vi "SIMUSIN.vi"() -> ()   [LabVIEW 2017]
uses:
  Typedefs/Tipo_TipoSinalSimulado.ctl
  Typedefs/Tipo_DadosCanal.ctl
  Typedefs/Tipo_BlocoSinais.ctl
  Typedefs/Tipo_ConfigSistema.ctl
  Typedefs/Tipo_ParamsRuido.ctl
  <vilib>/NI/STM/SubVIs/MetaDataElement.ctl
  <vilib>/NI/STM/Connection Manager/TCP/TCP Connection Method.ctl
  <vilib>/NI/STM/TCP/TCP Read Options.ctl
  Typedefs/Tipo_PoolComando.ctl
  <vilib>/NI/STM/TCP/Write Meta Data (TCP Ref).vi
  <vilib>/NI/STM/TCP/Write Meta Data (TCP Clst).vi
  <vilib>/NI/STM/TCP/Read Message (TCP).vi
  <vilib>/NI/STM/TCP/Write Message (TCP).vi
  <vilib>/NI/STM/TCP/TCP Connection Info.ctl
  <vilib>/NI/STM/NI STM.lvlib
panel:
  out "BlocoBaixaEnviado":i32
  out "SinaisBaixa":waveform(dbl)[](array[waveform])
  in  "ParamsCanalCopiado":variant
  out "DadosEstaticos":dbl[](array[numeric])
  in  "Tab Control":enum32{"Dinâmicos", "Estáticos"}(tab)
  in  "TxAmostragemBaixa":dbl=300.0 caption="Tx. Baixa (Hz):" min=50.0 max=50000.0
  out "NumConexoes":i32 caption="Num. Conexões"
  in  "CopiarCanal":bool
  in  "ColarCanal":bool
  in  "Canais":i32[](listbox)
  out "Índice":i32
  in  "Nome":string
  in  "Tipo":T1
  in  "NovoCanal":bool
  in  "AtualizarCanal":bool
  in  "ExcluirCanal":bool
  out "Frequência":cluster{"f0":dbl, "df":dbl, "magnitude":dbl[]}[](graph)
  out "Tempo":waveform(dbl)[](graph)
  in  "TxAmostragem":dbl=300.0 caption="Tx. Amostragem (Hz):" min=50.0 max=100000.0
  in  "Porta":u16=2099
  out "NumBloco":i32 caption="Bloco:"
  in  "SobeCanal":bool
  in  "DesceCanal":bool
  in  "Habilitar":bool caption="Habilitado"
  in  "Vizualizar Baixa":bool
  in  "Ver Fase":bool
  in  "RemoverPonto":bool
  in  "InserirPonto":bool
  in  "Sinais Estáticos":i32(listbox)
  in  "DesceCanalEstatico":bool
  in  "SobeCanalEstatico":bool
  out "Sinais":waveform(dbl)[](array[waveform])
  in  "ResetCanais":bool
  in  "Saiu?":bool
  in  "DadosCanais":T2[](array[typedef])
  # "SimuSinC - Simulador de Sinais"
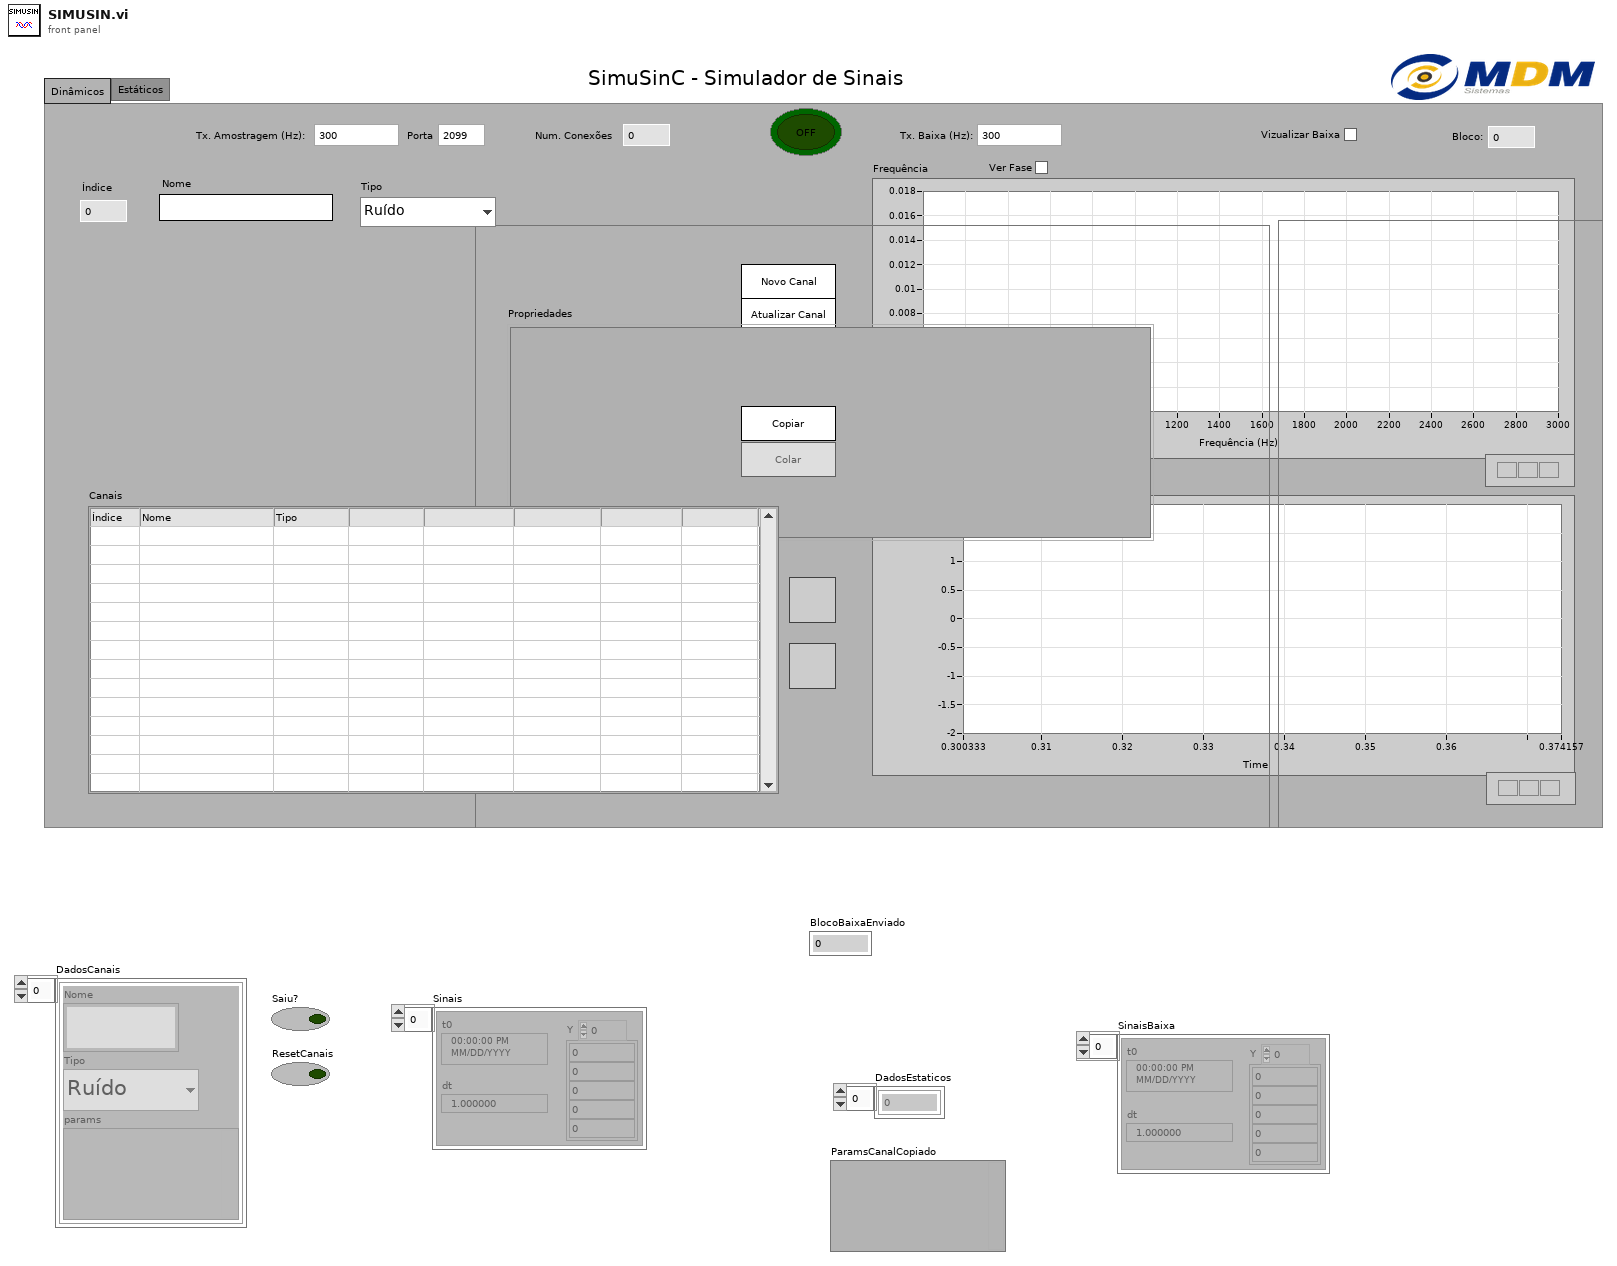
[diagram p1: front panel]
types:
  T1 = typedef "Tipo_TipoSinalSimulado.ctl" = enum16{"Ruído", "Fasor", "Senóide", "Composto", "AM", "Proximidade", "Entreferro"}
  T2 = typedef "Tipo_DadosCanal.ctl" = cluster{"Nome":string, "Tipo":T1, "params":variant}
  T3 = typedef "Tipo_BlocoSinais.ctl" = cluster{"SinaisAlta":waveform(dbl)[], "SinaisBaixa":waveform(dbl)[], "NumBloco":i32}
  T4 = enum8{"Enabled", "Disabled", "Disabled and Grayed Out"}
  T5 = typedef "Tipo_ConfigSistema.ctl" = cluster{"TxAmostragem":dbl, "Porta":u16, "TxAmostragemBaixa":dbl}
  T6 = typedef "Tipo_ParamsRuido.ctl" = cluster{"Amplitude":dbl, "Banda: ":bool, "Freq. Inferior":dbl, "Freq. Superior":dbl}
  T7 = typedef "FileVersionInformation.ctl" = cluster{"FileVersion":string, "ProductName":string, "InternalName":string, "CompanyName":string, "LegalCopyright":string, "FileDescription":string}
  T8 = typedef "LVPoint32TypeDef.ctl" = cluster{"Horizontal":i32, "Vertical":i32}
  T9 = typedef "LVRowAndColumnTypeDef.ctl" = cluster{"Row":i32, "Column":i32}
  T10 = typedef "NI STM.lvlib/TCP Connection Info.ctl" = cluster{"connection ID":refnum<k5>, "meta data":T11[]}
  T11 = typedef "NI STM.lvlib/MetaDataElement.ctl" = string
  T12 = typedef "Tipo_PoolComando.ctl" = enum16{"Indefinido", "ProximoBlocoAlta", "ProximoBlocoBaixa"}
  T13 = typedef "NI STM.lvlib/TCP Connection Method.ctl" = enum16{"Initialize", "Add Connection", "Set Properties", "Get Connection(s)", "Remove Connection", "Remove All Connections", "Get Connection Count"}
  T14 = typedef "NI STM.lvlib/TCP Read Options.ctl" = cluster{"ignore timeout error":bool, "timeout ms (1000)":i32}
  T15 = typedef "Tipo_PacoteModuloCRIO.ctl" = cluster{"modulo":T16, "sinais":cluster{"dados":sgl[]}[], "numBloco":i32}
  T16 = typedef "Tipo_moduloCRIO.ctl" = cluster{"nome":string, "modelo":string, "slot":i32, "numCanais":i32, "canaisInativos":i32[], "sensores":string[], "TaxaAquisicao":dbl}
  T17 = cluster{waveform(dbl)[], "SinaisBaixa":waveform(dbl)[], i32}
  T18 = enum32{"invalid app kind", "Development System", "Run Time System", "Student Edition", "Embedded LabVIEW", "Evaluation", "Custom"}
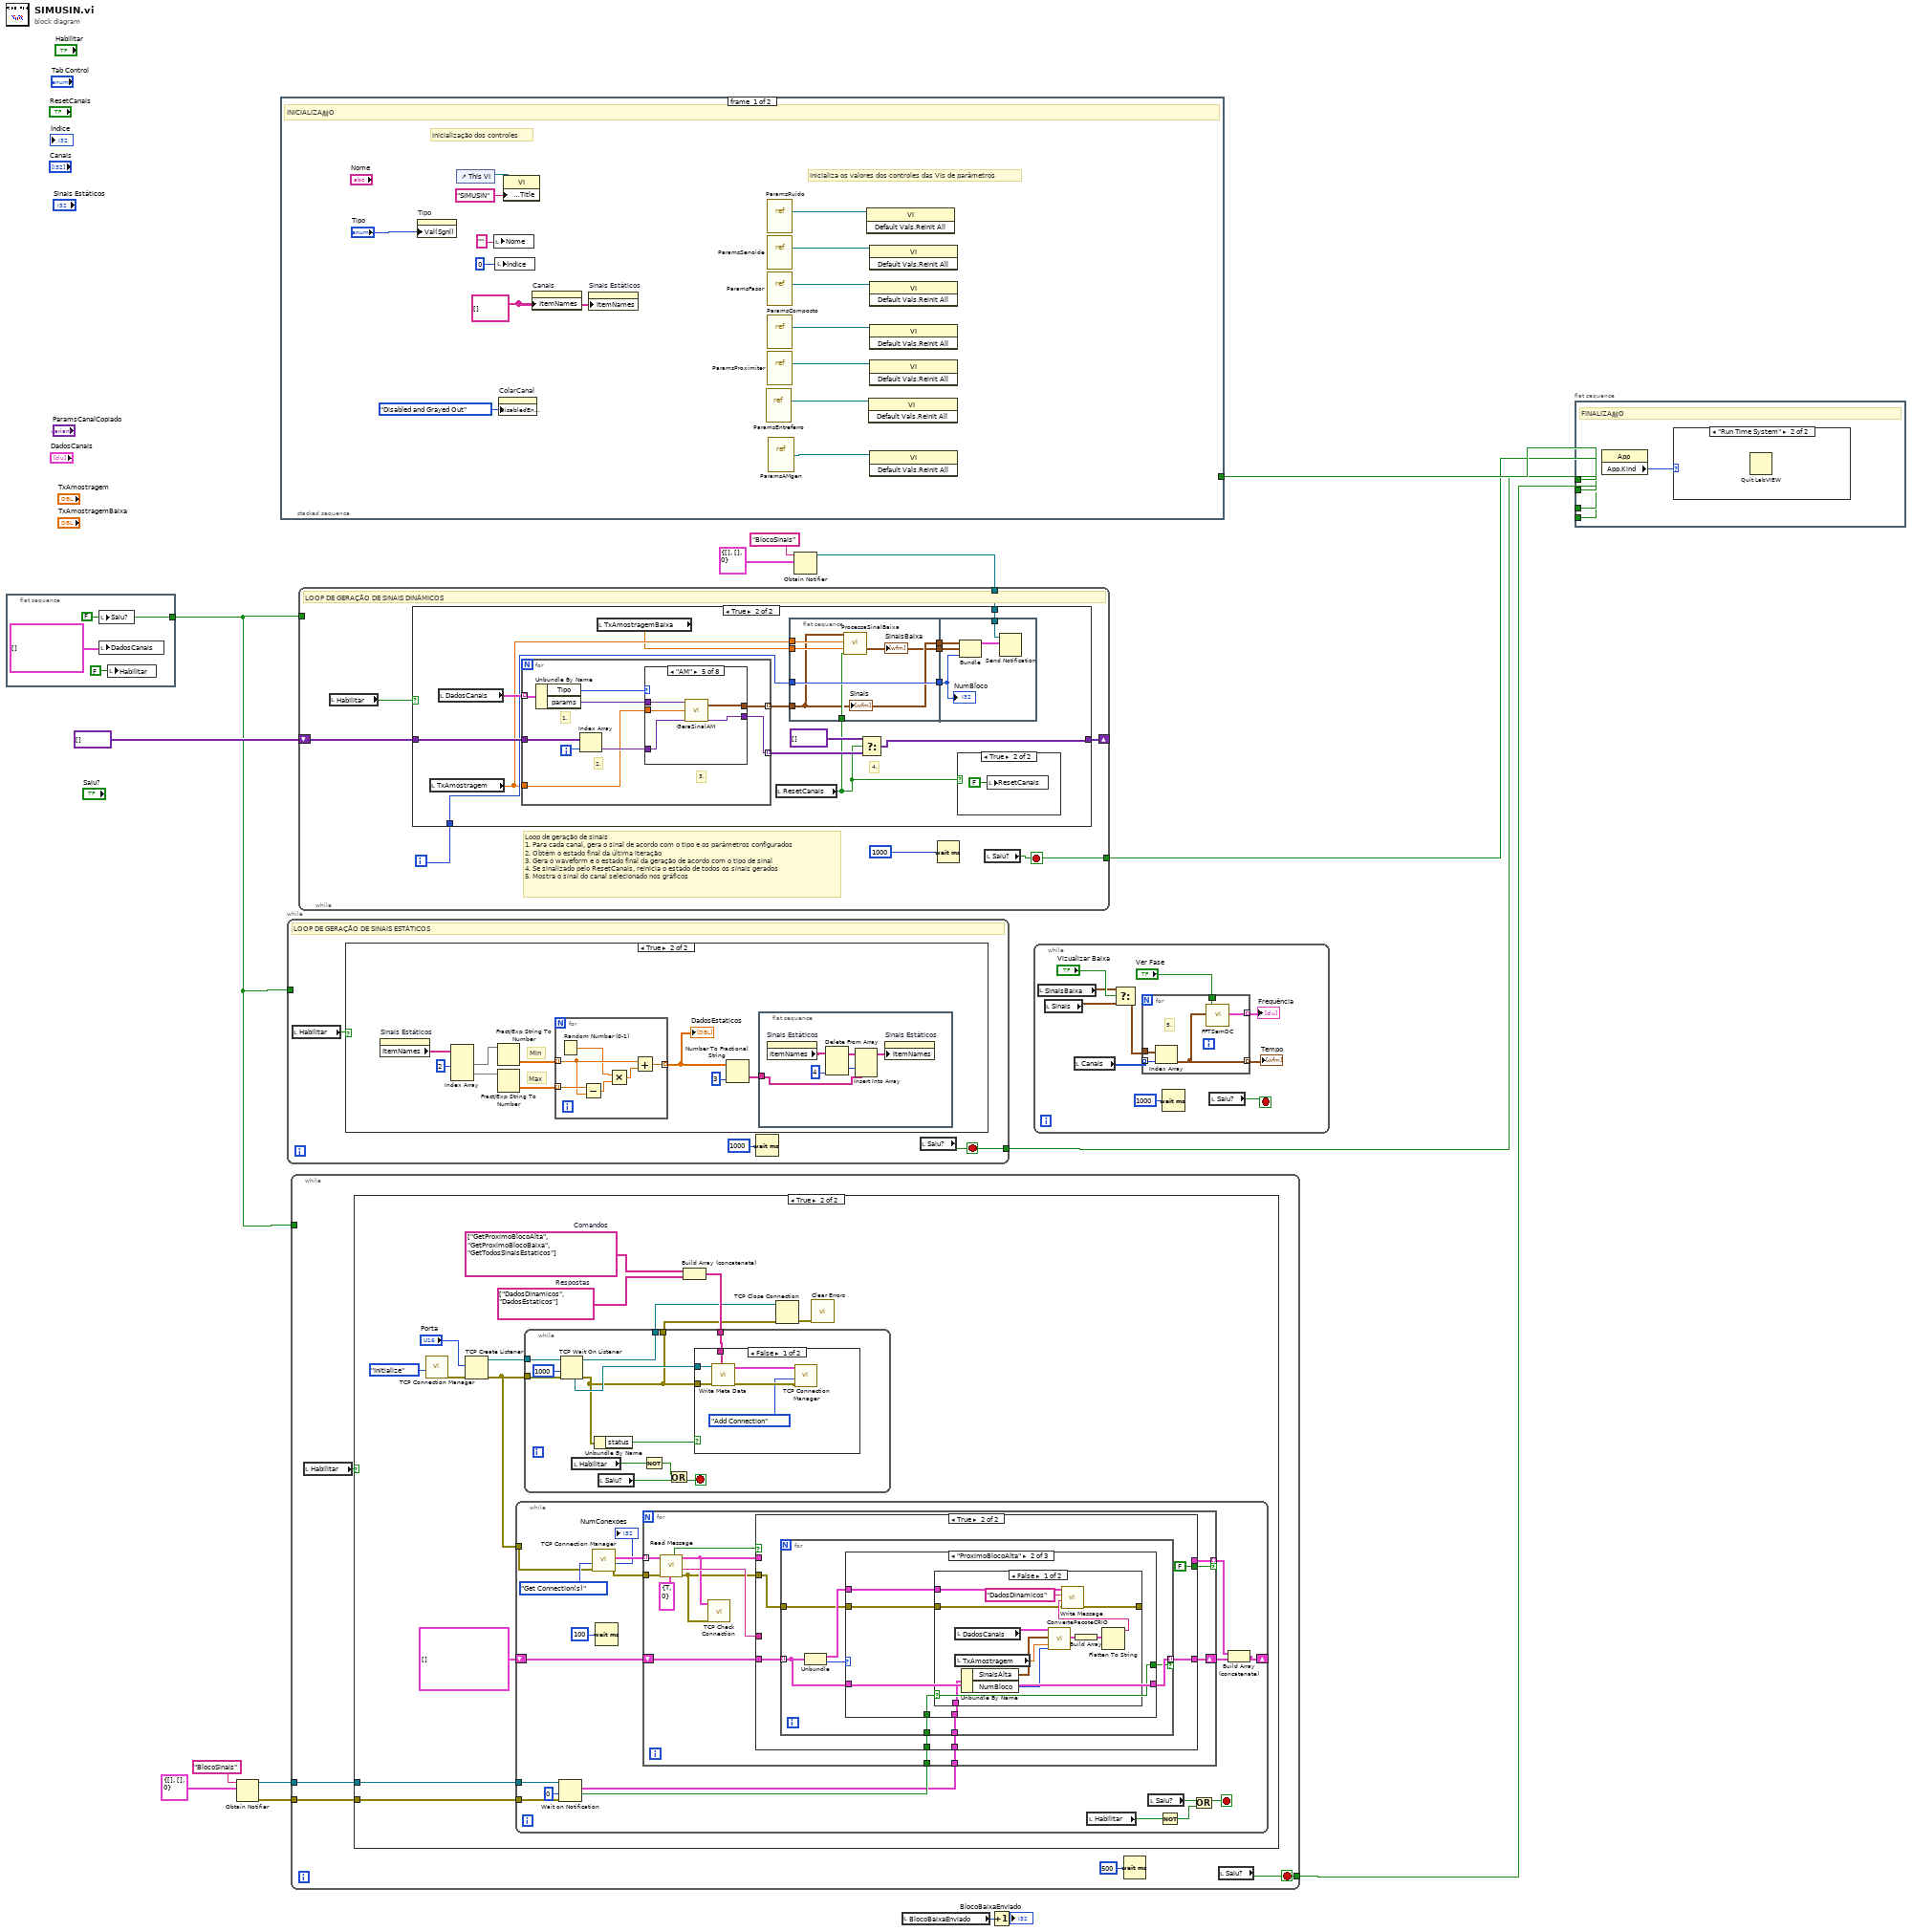
[diagram p0: block diagram]
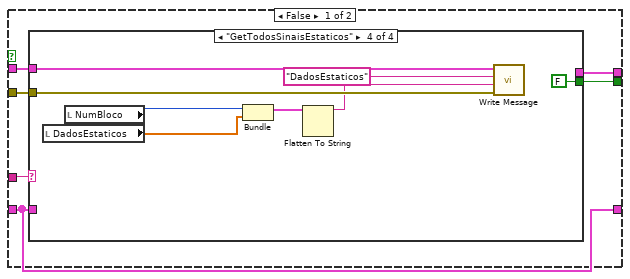
[diagram p3: hidden frame]
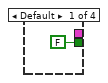
[diagram p4: hidden frame]
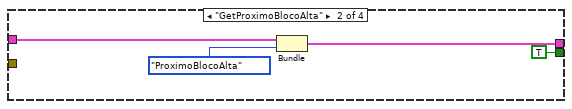
[diagram p5: hidden frame]
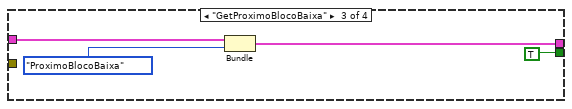
[diagram p6: hidden frame]
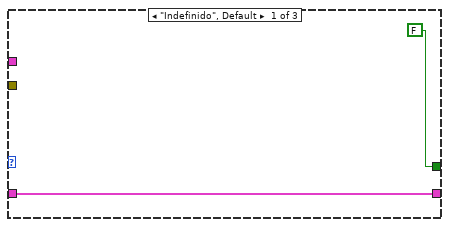
[diagram p7: hidden frame]
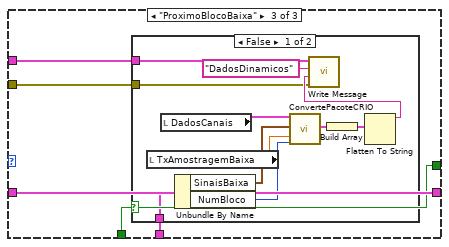
[diagram p9: hidden frame]
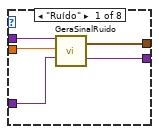
[diagram p16: hidden frame]
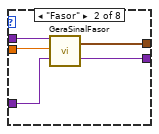
[diagram p17: hidden frame]
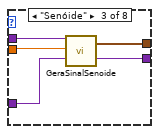
[diagram p18: hidden frame]
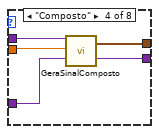
[diagram p19: hidden frame]
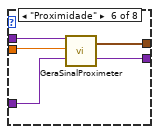
[diagram p20: hidden frame]
diagram:
  n1 = flat-sequence {
    tunnel: [w18] -> w10
    frame #0 {
      w18 = FALSE ("Saiu?")
      n2 = local write "Saiu?"(w18) -> ()
      n3 = local write "DadosCanais"(T2[] [] ("DadosCanais")) -> ()
      n4 = local write "Habilitar"(FALSE ("Habilitar")) -> ()
    }
  }
  n5 = Obtain Notifier(name (unnamed)="BlocoSinais", notification data type=T3 {"SinaisAlta"=[], "SinaisBaixa"=[], "NumBloco"=0} ("output cluster")) -> (notifier out=w4:refnum<notifier>, error out=w3:errorcluster)  [unwired: 2 in, 1 out]
  n6 = stacked-sequence {
    tunnel: [_ w33] -> w14
    frame #0 {
      w26 = string[][] [] ("Item Names")
      # "Inicializa os valores dos controles das VIs de parâmetros"
      # "Inicialização dos controles"
      # "INICIALIZA敲O"
      n7 = property on="Tipo" class="Enum (strict)"("Val(Sgnl)"="Tipo") -> ()  [unwired: 2 in, 2 out]
      n8 = control-ref of="This VI"() -> (w25:refnum<vi>)
      n9 = local write "Nome"("" ("Nome")) -> ()
      n10 = local write "Índice"(0 ("Índice")) -> ()
      n11 = property on="ColarCanal" class="Bool"("DisabledEnum"=T4."Disabled and Grayed Out" ("Disabled")) -> ()  [unwired: 2 in, 2 out]
      n12 = property class="VI"(reference=w25, "Front Panel.Title"="SIMUSIN" ("Front Panel Window:Title")) -> ()  [unwired: 1 in, 2 out]
      n13 = property on="Canais" class="MCListbox (strict)"("ItemNames"=w26) -> ()  [unwired: 2 in, 2 out]
      n14 = property on="Sinais Estáticos" class="MCListbox (strict)"("ItemNames"=w26) -> ()  [unwired: 2 in, 2 out]
      n15 = vi-ref "ParamsEntreferro.vi"() -> (w20:refnum<vi>)
      n16 = vi-ref "ParamsRuido.vi"() -> (w30:refnum<vi>)
      n17 = vi-ref "ParamsSenoide.vi"() -> (w29:refnum<vi>)
      n18 = vi-ref "ParamsFasor.vi"() -> (w28:refnum<vi>)
      n19 = vi-ref "ParamsComposto.vi"() -> (w21:refnum<vi>)
      n20 = vi-ref "ParamsProximiter.vi"() -> (w22:refnum<vi>)
      n21 = vi-ref "ParamsAMgen.vi"() -> (w19:refnum<vi>)
      n22 = invoke class="VI" method="Default Vals.Reinit All"(reference=w30) -> ()  [unwired: 2 in, 3 out]
      n23 = invoke class="VI" method="Default Vals.Reinit All"(reference=w20) -> ()  [unwired: 2 in, 3 out]
      n24 = invoke class="VI" method="Default Vals.Reinit All"(reference=w29) -> ()  [unwired: 2 in, 3 out]
      n25 = invoke class="VI" method="Default Vals.Reinit All"(reference=w28) -> ()  [unwired: 2 in, 3 out]
      n26 = invoke class="VI" method="Default Vals.Reinit All"(reference=w21) -> ()  [unwired: 2 in, 3 out]
      n27 = invoke class="VI" method="Default Vals.Reinit All"(reference=w22) -> ()  [unwired: 2 in, 3 out]
      n28 = invoke class="VI" method="Default Vals.Reinit All"(reference=w19) -> ()  [unwired: 2 in, 3 out]
    }
    frame #1 {
      # "LOOP DE INTERFACE"
      n29 = while {
        tunnel: [w34] -> w33
        stop <- w34 stop-if-true
        # "LOOP DE INTERFACE"
        n30 = event shown="[3] \"Tipo\": Value Change" {
          selector: _ -> [_ _ _ _ _ _ _ _ _ _ _ _ _ _ _ _ _ _ _]
          dyn-events: _ -> [_ _ _ _ _ _ _ _ _ _ _ _ _ _ _ _ _ _ _]
          timeout: 500 -> [_ _ _ _ _ _ _ _ _ _ _ _ _ _ _ _ _ _ _]
          tunnel: [_ _ w49 _ _ _ _ _ _ _ _ _ _ _ _ _ _ _ _] -> w34
          event Timeout {
            n31 = event-data() -> ()  [unwired: 1 in, 2 out]
          }
          event "Canais": Value Change {
            # "2."
            # "1."
            # "Evento: Troca de canal selecionado\n1. Obtém os dados do novo canal selecionado\n2. Muda o valor do tipo de sinal sinalizando o evento para atualizar o VI de parâmetros sendo mostrado\n3. Se for uma seleção válida, atualiza os parâmetros da VI apropriada\n4. Reinicia o chart do sinal no tempo"
            n32 = event-data() -> ("NewVal"=w41:i32[])  [unwired: 1 in, 4 out]
            n33 = Index Array(array=w41) -> (element=w36:i32)  [unwired: 1 in]
            n34 = local read "DadosCanais"() -> (w39:T2[])
            n35 = local write "Índice"(w36) -> ()
            n36 = Index Array(array=w39, index=w36) -> (element=w43:T2)
            n37 = Unbundle By Name(w43) -> ("Nome"=w42:string, "Tipo"=w37:T1, "params"=w40:variant)
            n38 = Array Size(array=w39) -> (size(s)=w38:i32)
            n39 = property on="Tipo" class="Enum (strict)"("Val(Sgnl)"=w37) -> ()  [unwired: 2 in, 2 out]
            n40 = local write "Nome"(w42) -> ()
            n41 = case shown="Default" w38 {
              tunnel: w40 -> [_ w46]
              tunnel: w37 -> [_ w45]
              frame 0 {
              }
              frame Default {
                # "3."
                n42 = call "GetVIParam.vi"("Tipo"=w45) -> ("vi reference"=w44:refnum<vi>)  [unwired: 18 in]
                n43 = call "AtualizaPainel.vi"("VI in"=w44, "Init"=TRUE, "ParamsIn"=w46) -> ()  [unwired: 16 in, 1 out]
              }
            }
          }
          event Menu Selection (User) {
            # "Processa eventos do menu superior"
            n44 = event-data() -> ("MenuRef"=w48:refnum<k9>, "ItemTag"=w50:string)  [unwired: 1 in, 4 out]
            n45 = case shown="\"ImportarDinamicos\"" w50 {
              selector: w50 -> [_ _ _ _ _ _ _ _ w170]
              tunnel: [FALSE TRUE _ FALSE FALSE FALSE FALSE FALSE _] -> w49
              tunnel: w48 -> [_ _ _ _ _ _ _ _ w171]
              frame Default {
              }
              frame "Sair" {
                # "Evento Sair"
              }
              frame "Sobre" {
                n46 = property class="App"() -> ("App.Dir"=w63:path, "App.Name"=w62:string)  [unwired: 2 in, 2 out]
                n47 = Build Path(base path=w63, name or relative path=w62) -> (appended path=w61:path)
                n48 = call <vilib>:"FileVersionInfo.vi"("Application Path in"=w61) -> ("FileVersionInfo Out"=w60:T7)  [unwired: 7 in, 3 out]
                n49 = Unbundle By Name(w60) -> ("ProductName"=w58:string, "FileVersion"=w57:string, "CompanyName"=w56:string, "LegalCopyright"=w55:string, "FileDescription"=w54:string)
                n50 = Format Into String(format string="%s versão %s\n%s\n%s\n%s", w58, w57, w56, w55, w54) -> (resulting string=w53:string)  [unwired: 2 in, 1 out]
                n51 = One Button Dialog(message=w53) -> ()  [unwired: 1 in, 1 out]
              }
              frame "SalvarConfig" {
                n52 = local read "TxAmostragemBaixa"() -> (w64:dbl)
                n53 = local read "TxAmostragem"() -> (w66:dbl)
                n54 = local read "Porta"() -> (w65:u16)
                n55 = call "File Dialog"("prompt"="Salvar arquivo de configuração", "pattern (all files)"="*.cfg", "pattern label"="Configuração de canais") -> ("selected path"=w73:path, "cancelled"=w71:bool, "error out"=w70:errorcluster)  [unwired: 9 in, 1 out]
                n56 = Bundle(cluster=T5 {"TxAmostragem"=0.0, "Porta"=0, "TxAmostragemBaixa"=0.0} ("output cluster"), "TxAmostragem"=w66, "Porta"=w65, "TxAmostragemBaixa"=w64) -> (w68:T5)
                n57 = case shown="False" w71 {
                  tunnel: w73 -> [w79 _]
                  tunnel: w70 -> [w77 _]
                  tunnel: w68 -> [w76 _]
                  frame False {
                    # "Salva os dados dos canais em arquivo"
                    n58 = local read "DadosCanais"() -> (w81:T2[])
                    n59 = property on="Sinais Estáticos" class="MCListbox (strict)"() -> ("ItemNames"=w80:string[][])  [unwired: 2 in, 2 out]
                    n60 = call "SalvarConfig.vi"("caminho in"=w79, "CanaisDinamicos"=w81, "CanaisEstaticos"=w80, "ConfigSistema"=w76, "error in"=w77) -> ("caminho out"=w78:path, "error out"=w82:errorcluster)  [unwired: 13 in]
                    n61 = case shown="No Error" w82 {
                      selector: w82 -> [_ w88]
                      tunnel: w78 -> [w83 _]
                      frame No Error {
                        n62 = Format Into String(format string="SIMUSIN (%s)", w83) -> (resulting string=w84:string)  [unwired: 2 in, 1 out]
                        n63 = control-ref of="This VI"() -> (w85:refnum<vi>)
                        n64 = property class="VI"(reference=w85, "Front Panel.Title"=w84) -> ()  [unwired: 1 in, 2 out]
                        n65 = One Button Dialog(message="Configuração salva com sucesso!") -> ()  [unwired: 1 in, 1 out]
                      }
                      frame Error {
                        n66 = call <vilib>:"Simple Error Handler.vi"("error in (no error)"=w88) -> ()  [unwired: 4 in, 5 out]
                      }
                    }
                  }
                  frame True {
                  }
                }
              }
              frame "CarregarConfig" {
                n67 = call "File Dialog2"("prompt"="Carregar arquivo de configuração", "pattern (all files)"="*.cfg", "pattern label"="Configuração de canais") -> ("selected path"=w92:path, "cancelled"=w91:bool, "error out"=w90:errorcluster)  [unwired: 9 in, 1 out]
                n68 = case shown="False" w91 {
                  tunnel: w92 -> [w109 _]
                  tunnel: w90 -> [w108 _]
                  frame False {
                    # "Carrega os dados dos canais\ndo arquivo"
                    n69 = call "CarregarConfig.vi"("caminho in"=w109, "error in (no error)"=w108) -> ("caminho out"=w106:path, "DadosCanais"=w110:T2[], "Estaticos"=w107:string[][], "ConfigSistema"=w105:T5, "error out"=w96:errorcluster)  [unwired: 13 in]
                    n70 = call <vilib>:"Simple Error Handler.vi"("error in (no error)"=w96) -> ()  [unwired: 4 in, 5 out]
                    n71 = Unbundle(w105) -> ("TxAmostragem"=w99:dbl, "Porta"=w98:u16, "TxAmostragemBaixa"=w97:dbl)
                    n72 = property on="Sinais Estáticos" class="MCListbox (strict)"("ItemNames"=w107) -> ()  [unwired: 2 in, 2 out]
                    n73 = Format Into String(format string="SIMUSIN (%s)", w106) -> (resulting string=w100:string)  [unwired: 2 in, 1 out]
                    n74 = local write "Porta"(w98) -> ()
                    n75 = local write "TxAmostragemBaixa"(w97) -> ()
                    n76 = local write "TxAmostragem"(w99) -> ()
                    n77 = call "PopulaListaCanais.vi"("DadosCanais"=w110) -> ("Strings"=w103:string[][])  [unwired: 18 in]
                    n78 = control-ref of="This VI"() -> (w102:refnum<vi>)
                    n79 = property on="Canais" class="MCListbox (strict)"("ItemNames"=w103) -> ()  [unwired: 2 in, 2 out]
                    n80 = local write "DadosCanais"(w110) -> ()
                    n81 = property class="VI"(reference=w102, "Front Panel.Title"=w100) -> ()  [unwired: 1 in, 2 out]
                    n82 = One Button Dialog(message="Configuração carregada com sucesso!") -> ()  [unwired: 1 in, 1 out]
                  }
                  frame True {
                  }
                }
              }
              frame "NovaConfig" {
                n83 = Two Button Dialog(message="Alterações não salvas na configuração atual\nserão perdidas. Deseja continuar? ", 1:"Não" ("T button name (\"OK\")"), 2:"Sim" ("T button name (\"OK\")")) -> (T button?=w112:bool)
                n84 = case shown="True" w112 {
                  frame False {
                  }
                  frame True {
                    n85 = local write "Nome"("" ("Nome")) -> ()
                    n86 = local write "Índice"(0 ("Índice")) -> ()
                    n87 = property on="Canais" class="MCListbox (strict)"("ItemNames"=string[][] [] ("Item Names")) -> ()  [unwired: 2 in, 2 out]
                    n88 = local write "DadosCanais"(T2[] [] ("DadosCanais")) -> ()
                  }
                }
              }
              frame "ImportarEstaticos" {
                n89 = call "File Dialog3"("pattern (all files)"="*.csv", "pattern label"="Arquivo CSV") -> ("selected path"=w121:path, "cancelled"=w122:bool, "error out"=w120:errorcluster)  [unwired: 10 in, 1 out]
                n90 = case shown="False" w122 {
                  tunnel: w121 -> [w141 _]
                  tunnel: w120 -> [w128 _]
                  frame False {
                    n91 = Read from Text File(file (use dialog)=w141, error in=w128) -> (text=w140:string, error out=w127:errorcluster)  [unwired: 2 in, 2 out]
                    n92 = Spreadsheet String To Array(delimiter (Tab)=";", format string="%s", spreadsheet string=w140, array type (2D Dbl)=string[][] []) -> (array=w133:string[][])
                    n93 = Array Size(array=w133) -> (size(s)=w136:i32[])
                    n94 = Index Array(array=w136) -> (element=w134:i32)  [unwired: 1 in]
                    n95 = Initialize Array("", w134) -> (w131:string[])
                    n96 = Insert Into Array(array=w133, index (col)=0 ("disabled index (col)"), new element=w131) -> (w130:string[][])  [unwired: 1 in]
                    n97 = call "IndexaEstaticos.vi"("Strings"=w130) -> ("StringsIndexadas"=w129:string[][])  [unwired: 18 in]
                    n98 = property on="Sinais Estáticos" class="MCListbox (strict)"(error in=w127, "ItemNames"=w129) -> (error out=w126:errorcluster)  [unwired: 1 in, 1 out]
                    n99 = case shown="No Error" w126 {
                      selector: w126 -> [_ w143]
                      frame No Error {
                        n100 = One Button Dialog(message="Arquivo importado com sucesso!") -> ()  [unwired: 1 in, 1 out]
                      }
                      frame Error {
                        n101 = call <vilib>:"Simple Error Handler.vi"("error in (no error)"=w143) -> ()  [unwired: 4 in, 5 out]
                      }
                    }
                  }
                  frame True {
                  }
                }
              }
              frame "ImportarDinamicos" {
                n102 = call "File Dialog4"("pattern (all files)"="*.csv", "pattern label"="Arquivo CSV") -> ("selected path"=w145:path, "cancelled"=w146:bool, "error out"=w144:errorcluster)  [unwired: 10 in, 1 out]
                n103 = case shown="False" w146 {
                  tunnel: w145 -> [w160 _]
                  tunnel: w144 -> [w155 _]
                  frame False {
                    n104 = Read from Text File(file (use dialog)=w160, error in=w155) -> (text=w159:string, error out=w151:errorcluster)  [unwired: 2 in, 2 out]
                    n105 = Spreadsheet String To Array(delimiter (Tab)=";", format string="%s", spreadsheet string=w159, array type (2D Dbl)=string[][] []) -> (array=w154:string[][])
                    n106 = for {
                      tunnel: w154 -> [w165] mode=indexing
                      tunnel: T2 {"Nome"="", "Tipo"=enum."Ruído", "params"=variant} -> [w166]
                      tunnel: [w163] -> w152 mode=indexing
                      n107 = Index Array(array=w165) -> (element=w164:string)  [unwired: 1 in]
                      n108 = Bundle By Name(cluster=w166, "Nome"=w164, "Tipo"=Tipo_TipoSinalSimulado."Senóide", "params"=T6 {"Amplitude"=0.0, "Banda: "=FALSE, "Freq. Inferior"=0.0, "Freq. Superior"=0.0} ("Tipo_ParamRuido")) -> (w163:T2)
                    }
                    n109 = call "PopulaListaCanais.vi"("DadosCanais"=w152) -> ("Strings"=w150:string[][])  [unwired: 18 in]
                    n110 = local write "DadosCanais"(w152) -> ()
                    n111 = property on="Canais" class="MCListbox (strict)"("ItemNames"=w150) -> ()  [unwired: 2 in, 2 out]
                    n112 = case shown="Error" w151 {
                      selector: w151 -> [_ w168]
                      frame No Error {
                        n113 = One Button Dialog(message="Arquivo importado com sucesso!") -> ()  [unwired: 1 in, 1 out]
                      }
                      frame Error {
                        n114 = call <vilib>:"Simple Error Handler.vi"("error in (no error)"=w168) -> ()  [unwired: 4 in, 5 out]
                      }
                    }
                  }
                  frame True {
                  }
                }
              }
              frame "FiltrarDecimar" {
                n115 = Get Menu Item Info(7:w170, 11:w171) -> (4:w169:bool)  [unwired: 1 in, 6 out]
                n116 = case shown="True" w169 {
                  frame False {
                  }
                  frame True {
                  }
                }
              }
            }
          }
          event Value Change {
            # "Mostra a VI de parâmetros no painel correspondente ao novo tipo de sinal selecionado"
            n117 = event-data() -> ("NewVal"=w173:T1)  [unwired: 1 in]
            n118 = call "GetVIParam.vi"("Tipo"=w173) -> ("vi reference"=w172:refnum<vi>)  [unwired: 18 in]
            n119 = invoke on="Propriedades" class="SubPanel" method="Insert VI"("VI Ref"=w172) -> ()  [unwired: 3 in, 4 out]
          }
          event "NovoCanal": Value Change {
            # "5."
            # "4."
            # "3."
            # "2."
            # "1."
            # "Evento: Novo canal criado\n1. Obtém os dados do painel como variant\n2. Monta o cluster de dados do canal\n3. Adiciona à lista de dados dos canais\n4. Atualiza a lista com todos os canais\n5. Reinicia a geração dos dados"
            n120 = event-data() -> ()  [unwired: 1 in, 1 out]
            n121 = property on="Propriedades" class="SubPnl"() -> ("InsertedVI"=w182:refnum<vi>)  [unwired: 2 in, 2 out]
            n122 = call "AtualizaPainel.vi"("VI in"=w182, "Init"=FALSE) -> ("ParamsOut"=w181:variant)  [unwired: 17 in]
            n123 = local read "Nome"() -> (w187:string)
            n124 = local read "Tipo"() -> (w186:T1)
            n125 = Bundle By Name(cluster=T2 {"Nome"="", "Tipo"=enum."Ruído", "params"=variant}, "params"=w181, "Nome"=w187, "Tipo"=w186) -> (w185:T2)
            n126 = local read "DadosCanais"() -> (w189:T2[])
            n127 = Insert Into Array(array=w189, new element=w185) -> (w184:T2[])  [unwired: 1 in]
            n128 = local write "DadosCanais"(w184) -> ()
            n129 = call "PopulaListaCanais.vi"("DadosCanais"=w184) -> ("Strings"=w183:string[][])  [unwired: 18 in]
            n130 = Array Size(array=w183) -> (size(s)=w177:i32[])
            n131 = Index Array(array=w177) -> (element=w178:i32)  [unwired: 1 in]
            n132 = Decrement(x=w178) -> (x-1=w175:i32)
            n133 = Build Array(w175) -> (w174:i32[])
            n134 = property on="Canais" class="MCListbox (strict)"("ItemNames"=w183, "Val(Sgnl)"=w174) -> (error out=w176:errorcluster)  [unwired: 2 in, 1 out]
            n135 = call <vilib>:"Clear Errors.vi"("error in (no error)"=w176) -> ()  [unwired: 5 in, 2 out]
            n136 = local write "ResetCanais"(TRUE ("ResetCanais")) -> ()
          }
          event "AtualizarCanal": Value Change {
            # "5."
            # "4."
            # "3."
            # "2."
            # "1."
            # "Evento: Canal atualizado\n1. Obtém os dados do painel como variant\n2. Monta o cluster de dados do canal\n3. Substitui o elemento no vetor de dados dos canais\n4. Atualiza a lista com todos os canais\n5. Reinicia a geração dos dados"
            n137 = event-data() -> ()  [unwired: 1 in, 1 out]
            n138 = property on="Propriedades" class="SubPnl"() -> ("InsertedVI"=w198:refnum<vi>)  [unwired: 2 in, 2 out]
            n139 = call "AtualizaPainel.vi"("VI in"=w198, "Init"=FALSE) -> ("ParamsOut"=w197:variant)  [unwired: 17 in]
            n140 = local read "Nome"() -> (w200:string)
            n141 = local read "Tipo"() -> (w199:T1)
            n142 = local read "Índice"() -> (w194:i32)
            n143 = local read "DadosCanais"() -> (w195:T2[])
            n144 = Bundle By Name(cluster=T2 {"Nome"="", "Tipo"=enum."Ruído", "params"=variant}, "params"=w197, "Nome"=w200, "Tipo"=w199) -> (w193:T2)
            n145 = Replace Array Subset(array=w195, new element=w193, index=w194) -> (w191:T2[])
            n146 = local write "DadosCanais"(w191) -> ()
            n147 = call "PopulaListaCanais.vi"("DadosCanais"=w191) -> ("Strings"=w192:string[][])  [unwired: 18 in]
            n148 = property on="Canais" class="MCListbox (strict)"("ItemNames"=w192) -> ()  [unwired: 2 in, 2 out]
            n149 = local write "ResetCanais"(TRUE ("ResetCanais")) -> ()
          }
          event "ExcluirCanal": Value Change {
            # "4."
            # "3."
            # "2."
            # "1."
            # "Evento: Canal excluído\n1. Remove o elemento da lista de dados dos canais\n2. Atualiza a lista de canais\n3. Seleciona o primeiro elemento  da lista de canais (gerando evento)\n4. Reinicia a geração de dados"
            n150 = event-data() -> ()  [unwired: 1 in, 1 out]
            n151 = local read "DadosCanais"() -> (w212:T2[])
            n152 = local read "Índice"() -> (w206:i32)
            n153 = Delete From Array(array=w212, index=w206) -> (array with subset deleted=w211:T2[])  [unwired: 1 in, 1 out]
            n154 = local write "DadosCanais"(w211) -> ()
            n155 = call "PopulaListaCanais.vi"("DadosCanais"=w211) -> ("Strings"=w209:string[][])  [unwired: 18 in]
            n156 = property on="Canais" class="MCListbox (strict)"("ItemNames"=w209) -> ()  [unwired: 2 in, 2 out]
            n157 = Array Size(array=w209) -> (size(s)=w208:i32[])
            n158 = Index Array(array=w208) -> (element=w207:i32)  [unwired: 1 in]
            n159 = Greater?(x=w207, y=w206) -> (0:w205:bool)
            n160 = Build Array(w206) -> (w204:i32[])
            n161 = Select(t=w204, s=w205, f=i32[] []) -> (s? t:f=w202:i32[])
            n162 = property on="Canais" class="MCListbox (strict)"("Val(Sgnl)"=w202) -> ()  [unwired: 2 in, 2 out]
            n163 = local write "ResetCanais"(TRUE ("ResetCanais")) -> ()
          }
          event "CopiarCanal": Value Change {
            n164 = event-data() -> ()  [unwired: 1 in, 1 out]
            n165 = property on="Propriedades" class="SubPnl"() -> ("InsertedVI"=w216:refnum<vi>)  [unwired: 2 in, 2 out]
            n166 = call "AtualizaPainel.vi"("VI in"=w216, "Init"=FALSE) -> ("ParamsOut"=w214:variant)  [unwired: 17 in]
            n167 = local write "ParamsCanalCopiado"(w214) -> ()
            n168 = property on="ColarCanal" class="Bool"("DisabledEnum"=T4."Enabled" ("Disabled")) -> ()  [unwired: 2 in, 2 out]
          }
          event "ColarCanal": Value Change {
            n169 = event-data() -> ()  [unwired: 1 in, 1 out]
            n170 = local read "ParamsCanalCopiado"() -> (w217:variant)
            n171 = property on="Propriedades" class="SubPnl"() -> ("InsertedVI"=w219:refnum<vi>)  [unwired: 2 in, 2 out]
            n172 = call "AtualizaPainel.vi"("VI in"=w219, "Init"=TRUE, "ParamsIn"=w217) -> ()  [unwired: 16 in, 1 out]
          }
          event "SobeCanal": Value Change {
            n173 = event-data() -> ()  [unwired: 1 in, 1 out]
            n174 = local read "Canais"() -> (w221:i32[])
            n175 = Index Array(array=w221) -> (element=w220:i32)  [unwired: 1 in]
            n176 = Greater Than 0?(x=w220) -> (x > 0?=w222:bool)
            n177 = case shown="True" w222 {
              tunnel: w220 -> [_ w227]
              frame False {
              }
              frame True {
                n178 = local read "DadosCanais"() -> (w230:T2[])
                n179 = Delete From Array(array=w230, index=w227) -> (deleted portion=w228:T2, array with subset deleted=w229:T2[])  [unwired: 1 in]
                n180 = Decrement(x=w227) -> (x-1=w224:i32)
                n181 = Build Array(w224) -> (w223:i32[])
                n182 = Insert Into Array(array=w229, index=w224, new element=w228) -> (w225:T2[])
                n183 = local write "DadosCanais"(w225) -> ()
                n184 = call "PopulaListaCanais.vi"("DadosCanais"=w225) -> ("Strings"=w226:string[][])  [unwired: 18 in]
                n185 = property on="Canais" class="MCListbox (strict)"("ItemNames"=w226, "Val(Sgnl)"=w223) -> ()  [unwired: 2 in, 2 out]
              }
            }
          }
          event "DesceCanal": Value Change {
            n186 = event-data() -> ()  [unwired: 1 in, 1 out]
            n187 = local read "Canais"() -> (w236:i32[])
            n188 = local read "DadosCanais"() -> (w235:T2[])
            n189 = Index Array(array=w236) -> (element=w231:i32)  [unwired: 1 in]
            n190 = Array Size(array=w235) -> (size(s)=w234:i32)
            n191 = Decrement(x=w234) -> (x-1=w233:i32)
            n192 = Less?(x=w231, y=w233) -> (x < y?=w232:bool)
            n193 = case shown="True" w232 {
              tunnel: w231 -> [_ w242]
              tunnel: w235 -> [_ w238]
              frame False {
              }
              frame True {
                n194 = Delete From Array(array=w238, index=w242) -> (deleted portion=w243:T2, array with subset deleted=w244:T2[])  [unwired: 1 in]
                n195 = Increment(x=w242) -> (x+1=w239:i32)
                n196 = Insert Into Array(array=w244, index=w239, new element=w243) -> (w240:T2[])
                n197 = Build Array(w239) -> (w237:i32[])
                n198 = call "PopulaListaCanais.vi"("DadosCanais"=w240) -> ("Strings"=w241:string[][])  [unwired: 18 in]
                n199 = local write "DadosCanais"(w240) -> ()
                n200 = property on="Canais" class="MCListbox (strict)"("ItemNames"=w241, "Val(Sgnl)"=w237) -> ()  [unwired: 2 in, 2 out]
              }
            }
          }
          event "Habilitar": Value Change {
            n201 = event-data() -> ()  [unwired: 1 in, 1 out]
          }
          event "Sinais Estáticos": Double Click {
            n202 = event-data() -> ("Coords"=w247:T8)  [unwired: 1 in]
            n203 = invoke on="Sinais Estáticos" class="MCListbox (strict)" method="Point To Row Column"("Point"=w247) -> ("CellPosition"=w245:T9)  [unwired: 6 in, 6 out]
            n204 = Unbundle(w245) -> ("Column"=w246:i32)  [unwired: 1 out]
            n205 = case shown="1..3" w246 {
              tunnel: w245 -> [_ w248]
              frame Default {
              }
              frame 1..3 {
                n206 = property on="Sinais Estáticos" class="MCListbox (strict)"("EditPos"=w248) -> ()  [unwired: 2 in, 2 out]
              }
            }
          }
          event "Sinais Estáticos": Edit Cell? {
            n207 = event-data() -> ("String"=w253:string, "Coords"=w251:T9)  [unwired: 1 in]
            n208 = invoke on="Sinais Estáticos" class="MCListbox (strict)" method="Point To Row Column"("Point"=w251) -> ("CellPosition"=w250:T9)  [unwired: 6 in, 6 out]
            n209 = Unbundle By Name(w250) -> ("Column"=w249:i32)
            n210 = case shown="2, 3" w249 {
              tunnel: w253 -> [w254 w263]
              tunnel: [w254 w261] -> w252
              frame Default {
              }
              frame 2, 3 {
                n211 = Fract/Exp String To Number(string=w263) -> (number=w256:dbl)  [unwired: 3 in, 1 out]
                n212 = In Range and Coerce(upper limit=inf, x=w256, lower limit=-inf) -> (In Range?=w258:bool)  [unwired: 1 out]
                n213 = Select(t=w256, s=w258, f=0.0) -> (s? t:f=w255:dbl)
                n214 = Format Into String(format string="%.3f", w255) -> (resulting string=w261:string)  [unwired: 2 in, 1 out]
              }
            }
            n215 = event-data("String"=w252) -> ()  [unwired: 2 in, 1 out]
          }
          event "Sinais Estáticos": Edit Cell {
            n216 = event-data() -> ()  [unwired: 1 in, 1 out]
            n217 = property on="Sinais Estáticos" class="MCListbox (strict)"() -> ("ItemNames"=w265:string[][])  [unwired: 2 in, 2 out]
            n218 = call "IndexaEstaticos.vi"("Strings"=w265) -> ("StringsIndexadas"=w264:string[][])  [unwired: 18 in]
            n219 = property on="Sinais Estáticos" class="MCListbox (strict)"("ItemNames"=w264) -> ()  [unwired: 2 in, 2 out]
          }
          event "InserirPonto": Value Change {
            w271 = "0" ("element")
            n220 = event-data() -> ()  [unwired: 1 in, 1 out]
            n221 = local read "Sinais Estáticos"() -> (w273:i32)
            n222 = property on="Sinais Estáticos" class="MCListbox (strict)"() -> ("ItemNames"=w274:string[][])  [unwired: 2 in, 2 out]
            n223 = Increment(x=w273) -> (x+1=w266:i32)
            n224 = Number To Decimal String(number=w266) -> (decimal integer string=w272:string)  [unwired: 1 in]
            n225 = Build Array(w272, "Novo Ponto" ("element"), w271, w271) -> (w269:string[])
            n226 = Insert Into Array(array=w274, index (row)=w266, new element=w269) -> (w268:string[][])  [unwired: 1 in]
            n227 = call "IndexaEstaticos.vi"("Strings"=w268) -> ("StringsIndexadas"=w267:string[][])  [unwired: 18 in]
            n228 = property on="Sinais Estáticos" class="MCListbox (strict)"("ItemNames"=w267) -> ()  [unwired: 2 in, 2 out]
          }
          event "RemoverPonto": Value Change {
            n229 = event-data() -> ()  [unwired: 1 in, 1 out]
            n230 = local read "Sinais Estáticos"() -> (w277:i32)
            n231 = property on="Sinais Estáticos" class="MCListbox (strict)"() -> ("ItemNames"=w278:string[][])  [unwired: 2 in, 2 out]
            n232 = Delete From Array(array=w278, index (row)=w277) -> (array with subset deleted=w276:string[][])  [unwired: 2 in, 1 out]
            n233 = call "IndexaEstaticos.vi"("Strings"=w276) -> ("StringsIndexadas"=w275:string[][])  [unwired: 18 in]
            n234 = property on="Sinais Estáticos" class="MCListbox (strict)"("ItemNames"=w275) -> ()  [unwired: 2 in, 2 out]
          }
          event "SobeCanalEstatico": Value Change {
            n235 = event-data() -> ()  [unwired: 1 in, 1 out]
            n236 = local read "Sinais Estáticos"() -> (w282:i32)
            n237 = property on="Sinais Estáticos" class="MCListbox (strict)"() -> ("ItemNames"=w285:string[][])  [unwired: 2 in, 2 out]
            n238 = Delete From Array(array=w285, index (row)=w282) -> (deleted portion=w283:string[], array with subset deleted=w284:string[][])  [unwired: 2 in]
            n239 = Decrement(x=w282) -> (x-1=w279:i32)
            n240 = Insert Into Array(array=w284, index (row)=w279, new element=w283) -> (w281:string[][])  [unwired: 1 in]
            n241 = local write "Sinais Estáticos"(w279) -> ()
            n242 = call "IndexaEstaticos.vi"("Strings"=w281) -> ("StringsIndexadas"=w280:string[][])  [unwired: 18 in]
            n243 = property on="Sinais Estáticos" class="MCListbox (strict)"("ItemNames"=w280) -> ()  [unwired: 2 in, 2 out]
          }
          event "DesceCanalEstatico": Value Change {
            n244 = event-data() -> ()  [unwired: 1 in, 1 out]
            n245 = local read "Sinais Estáticos"() -> (w289:i32)
            n246 = property on="Sinais Estáticos" class="MCListbox (strict)"() -> ("ItemNames"=w292:string[][])  [unwired: 2 in, 2 out]
            n247 = Delete From Array(array=w292, index (row)=w289) -> (deleted portion=w290:string[], array with subset deleted=w291:string[][])  [unwired: 2 in]
            n248 = Increment(x=w289) -> (x+1=w286:i32)
            n249 = Insert Into Array(array=w291, index (row)=w286, new element=w290) -> (w288:string[][])  [unwired: 1 in]
            n250 = local write "Sinais Estáticos"(w286) -> ()
            n251 = call "IndexaEstaticos.vi"("Strings"=w288) -> ("StringsIndexadas"=w287:string[][])  [unwired: 18 in]
            n252 = property on="Sinais Estáticos" class="MCListbox (strict)"("ItemNames"=w287) -> ()  [unwired: 2 in, 2 out]
          }
        }
        n253 = local write "Saiu?"(w34) -> ()
      }
    }
  }
  n254 = while {
    tunnel: [w295] -> w12
    tunnel: w10 -> [_]
    stop <- w295 stop-if-true
    # "LOOP DE GERAÇÃO DE SINAIS ESTÁTICOS"
    n255 = local read "Habilitar"() -> (w293:bool)
    n256 = case shown="True" w293 {
      frame False {
      }
      frame True {
        # "Max"
        # "Min"
        n257 = property on="Sinais Estáticos" class="MCListbox (strict)"() -> ("ItemNames"=w304:string[][])  [unwired: 2 in, 2 out]
        n258 = Index Array(array=w304, index (col) #1=2 ("disabled index (col)")) -> (element #1=w302:string[], element #2=w301:string[])  [unwired: 3 in]
        n259 = Fract/Exp String To Number(string=w302) -> (number=w300:dbl[])  [unwired: 3 in, 1 out]
        n260 = Fract/Exp String To Number(string=w301) -> (number=w299:dbl[])  [unwired: 3 in, 1 out]
        n261 = for {
          tunnel: w300 -> [w314] mode=indexing
          tunnel: w299 -> [w315] mode=indexing
          tunnel: [w310] -> w298 mode=indexing
          n262 = Random Number (0-1)() -> (number: 0 to 1=w312:dbl)
          n263 = Subtract(x=w315, y=w314) -> (x-y=w313:dbl)
          n264 = Multiply(x=w312, y=w313) -> (x*y=w311:dbl)
          n265 = Add(x=w314, y=w311) -> (x+y=w310:dbl)
        }
        "DadosEstaticos" <- w298
        n266 = Number To Fractional String(number=w298, precision (6)=i16 3) -> (F-format string=w296:string[])  [unwired: 2 in]
        n267 = flat-sequence {
          tunnel: w296 -> [w307]
          frame #0 {
            w306 = 4 ("disabled index (col)")
            n268 = property on="Sinais Estáticos" class="MCListbox (strict)"() -> ("ItemNames"=w309:string[][])  [unwired: 2 in, 2 out]
            n269 = Delete From Array(array=w309, index (col)=w306) -> (array with subset deleted=w308:string[][])  [unwired: 2 in, 1 out]
            n270 = Insert Into Array(array=w308, index (col)=w306, new element=w307) -> (w305:string[][])  [unwired: 1 in]
            n271 = property on="Sinais Estáticos" class="MCListbox (strict)"("ItemNames"=w305) -> ()  [unwired: 2 in, 2 out]
          }
        }
      }
    }
    n272 = Wait (ms)(milliseconds to wait=u32 1000) -> ()  [unwired: 1 out]
    n273 = local read "Saiu?"() -> (w295:bool)
  }
  n274 = while {
    tunnel: [w320] -> w11
    tunnel: w10 -> [_]
    tunnel: w4 -> [w317]
    tunnel: w3 -> [w316]
    stop <- w320 stop-if-true
    n275 = local read "Habilitar"() -> (w319:bool)
    n276 = case shown="True" w319 {
      tunnel: w317 -> [_ w322]
      tunnel: w316 -> [_ w321]
      frame False {
      }
      frame True {
        w329 = T11[] ["DadosDinamicos", "DadosEstaticos"]  # Respostas
        w332 = T11[] ["GetProximoBlocoAlta", "GetProximoBlocoBaixa", "GetTodosSinaisEstaticos"]  # Comandos
        n277 = call <vilib>:"TCP Connection Manager.vi"("method"=TCP_Connection_Method."Initialize") -> ("error out"=w333:errorcluster)  [unwired: 5 in, 5 out]
        n278 = TCP Create Listener(8:w333, 10:"Porta") -> (0:w328:errorcluster, 3:w334:refnum<k5>)  [unwired: 3 in, 1 out]
        n279 = while {
          tunnel: w328 -> [w350]
          shift-right: [w336] -> _
          shift-left: cluster{"connection info out":T10, T12}[] [] -> [w342]
          tunnel: w322 -> [w341]
          tunnel: w321 -> [w340]
          stop <- w348 stop-if-true
          n280 = Wait on Notification(notifier=w341, timeout in ms (-1)=0, error in (no error)=w340) -> (notification=w337:T3, timed out?=w338:bool)  [unwired: 1 in, 2 out]
          n281 = call <vilib>:"TCP Connection Manager.vi"("error in"=w350, "method"=TCP_Connection_Method."Get Connection(s)") -> ("error out"=w345:errorcluster, "number of connections"=→"NumConexoes":i32, "all connections"=w352:T10[])  [unwired: 4 in, 3 out]
          n282 = Wait (ms)(milliseconds to wait=u32 100) -> ()  [unwired: 1 out]
          n283 = for {
            tunnel: w352 -> [w366] mode=indexing
            tunnel: w345 -> [w360]
            shift-right: [w359] -> w343
            shift-left: w342 -> [w358]
            tunnel: w338 -> [w357]
            tunnel: w337 -> [w356]
            tunnel: [w355] -> w335 mode=indexing if=w354
            n284 = call-poly <vilib>:"Read Message.vi"("options"=T14 {"ignore timeout error"=TRUE, "timeout ms (1000)"=0}, "error in"=w360, "connection info in"=w366) -> ("error out"=w361:errorcluster, "name"=w363:T11, "connection info out"=w362:T10, "timed out?"=w364:bool)  [unwired: 3 in, 2 out]
            n285 = call <vilib>:"TCP Check Connection.vi"("error in"=w361, "connection in"=w362) -> ()  [unwired: 7 in, 3 out]
            n286 = case shown="True" w364 {
              tunnel: w363 -> [w370 _]
              tunnel: w362 -> [w372 _]
              tunnel: w361 -> [w371 w393]
              tunnel: [w369 w392] -> w359
              tunnel: w358 -> [w369 w395]
              tunnel: w357 -> [_ w394]
              tunnel: w356 -> [_ w391]
              tunnel: [w368 _] -> w355
              tunnel: [w367 FALSE] -> w354
              frame False {
                n287 = case shown="\"GetTodosSinaisEstaticos\"" w370 {
                  tunnel: w372 -> [_ w377 w381 w389]
                  tunnel: w371 -> [_ _ _ w388]
                  tunnel: [_ w375 w379 _] -> w368
                  tunnel: w369 -> [_ _ _ _]
                  tunnel: [FALSE TRUE TRUE FALSE] -> w367
                  frame Default {
                  }
                  frame "GetProximoBlocoAlta" {
                    n288 = Bundle("connection info out"=w377, Tipo_PoolComando."ProximoBlocoAlta") -> (w375:cluster{"connection info out":T10, T12})  [unwired: 1 in]
                  }
                  frame "GetProximoBlocoBaixa" {
                    n289 = Bundle("connection info out"=w381, Tipo_PoolComando."ProximoBlocoBaixa") -> (w379:cluster{"connection info out":T10, T12})  [unwired: 1 in]
                  }
                  frame "GetTodosSinaisEstaticos" {
                    n290 = local read "DadosEstaticos"() -> (w384:dbl[])
                    n291 = local read "NumBloco"() -> (w385:i32)
                    n292 = Bundle("NumBloco"=w385, "DadosEstaticos"=w384) -> (w383:cluster{"NumBloco":i32, "DadosEstaticos":dbl[]})  [unwired: 1 in]
                    n293 = Flatten To String(anything=w383) -> (data string=w387:string)  [unwired: 3 in, 2 out]
                    n294 = call-poly <vilib>:"Write Message.vi"("error in"=w388, "data"=w387, "name"="DadosEstaticos", "connection info in"=w389) -> ()  [unwired: 6 in, 2 out]
                  }
                }
              }
              frame True {
                n295 = for {
                  tunnel: w395 -> [w399] mode=indexing
                  tunnel: w394 -> [w402]
                  tunnel: w393 -> [w400]
                  tunnel: [w398] -> w392 mode=indexing if=w397
                  tunnel: w391 -> [w396]
                  n296 = Unbundle(w399) -> ("connection info out"=w401:T10, w403:T12)
                  n297 = case shown="\"ProximoBlocoAlta\"" w403 {
                    tunnel: w402 -> [_ w407 w424]
                    tunnel: w401 -> [_ w410 w427]
                    tunnel: w400 -> [_ w409 w426]
                    tunnel: w399 -> [w405 w408 w425]
                    tunnel: [w405 w408 w425] -> w398
                    tunnel: [FALSE w407 w424] -> w397
                    tunnel: w396 -> [_ w406 w423]
                    frame "Indefinido", Default {
                    }
                    frame "ProximoBlocoAlta" {
                      n298 = case shown="False" w407 {
                        tunnel: w410 -> [w418 _]
                        tunnel: w409 -> [w415 _]
                        tunnel: [w414 _] -> _
                        tunnel: w406 -> [w413 _]
                        frame False {
                          n299 = local read "DadosCanais"() -> (w422:T2[])
                          n300 = local read "TxAmostragem"() -> (w421:dbl)
                          n301 = Unbundle By Name(w413) -> ("SinaisAlta"=w411:waveform(dbl)[], "NumBloco"=w412:i32)
                          n302 = call "ConvertePacoteCRIO.vi"("DadosCanais"=w422, "Sinais"=w411, "Tx Aquisicao"=w421, "numBloco"=w412) -> ("Tipo_PacoteModuloCRIO"=w420:T15)  [unwired: 15 in]
                          n303 = Build Array(w420) -> (w419:T15[])
                          n304 = Flatten To String(anything=w419) -> (data string=w416:string)  [unwired: 3 in, 2 out]
                          n305 = call-poly <vilib>:"Write Message.vi"("error in"=w415, "data"=w416, "name"="DadosDinamicos", "connection info in"=w418) -> ("error out"=w414:errorcluster)  [unwired: 6 in, 1 out]
                        }
                        frame True {
                        }
                      }
                    }
                    frame "ProximoBlocoBaixa" {
                      n306 = case shown="False" w424 {
                        tunnel: w427 -> [w434 _]
                        tunnel: w426 -> [w431 _]
                        tunnel: w423 -> [w430 _]
                        frame False {
                          n307 = local read "TxAmostragemBaixa"() -> (w437:dbl)
                          n308 = local read "DadosCanais"() -> (w438:T2[])
                          n309 = Unbundle By Name(w430) -> ("SinaisBaixa"=w429:waveform(dbl)[], "NumBloco"=w428:i32)
                          n310 = call "ConvertePacoteCRIO.vi"("DadosCanais"=w438, "Sinais"=w429, "Tx Aquisicao"=w437, "numBloco"=w428) -> ("Tipo_PacoteModuloCRIO"=w436:T15)  [unwired: 15 in]
                          n311 = Build Array(w436) -> (w435:T15[])
                          n312 = Flatten To String(anything=w435) -> (data string=w432:string)  [unwired: 3 in, 2 out]
                          n313 = call-poly <vilib>:"Write Message.vi"("error in"=w431, "data"=w432, "name"="DadosDinamicos", "connection info in"=w434) -> ()  [unwired: 6 in, 2 out]
                        }
                        frame True {
                        }
                      }
                    }
                  }
                }
              }
            }
          }
          n314 = local read "Habilitar"() -> (w347:bool)
          n315 = local read "Saiu?"() -> (w351:bool)
          n316 = Not(x=w347) -> (.not. x?=w346:bool)
          n317 = Or(x=w351, y=w346) -> (x .or. y?=w348:bool)
          n318 = Build Array (concatenate)(w335, w343) -> (w336:cluster{"connection info out":T10, T12}[])
        }
        n319 = Build Array (concatenate)(w332, w329) -> (w330:T11[])
        n320 = while "Listen loop.  Append new connections to a synchronized queue." {
          tunnel: w334 -> [w449]
          tunnel: w328 -> [w450]
          tunnel: w330 -> [w447]
          tunnel: [w440] -> w326
          tunnel: [w439] -> w324
          stop <- w444 stop-if-true
          n321 = TCP Wait On Listener(8:w450, 9:1000 ("timeout ms (wait forever: -1)"), 11:w449) -> (0:w440:errorcluster, 3:w439:refnum<k5>, 4:w441:refnum<k5>)  [unwired: 1 in, 2 out]
          n322 = local read "Habilitar"() -> (w443:bool)
          n323 = Unbundle By Name(w440) -> ("status"=w448:bool)
          n324 = local read "Saiu?"() -> (w445:bool)
          n325 = Not(x=w443) -> (.not. x?=w442:bool)
          n326 = Or(x=w442, y=w445) -> (x .or. y?=w444:bool)
          n327 = case shown="False" w448 {
            tunnel: w441 -> [w456 _]
            tunnel: w440 -> [w455 _]
            tunnel: w447 -> [w454 _]
            frame False {
              n328 = call-poly <vilib>:"Write Meta Data.vi"("meta data"=w454, "error in"=w455, "connection ID"=w456) -> ("error out"=w452:errorcluster, "connection info out"=w453:T10)  [unwired: 7 in]
              n329 = call <vilib>:"TCP Connection Manager.vi"("error in"=w452, "method"=TCP_Connection_Method."Add Connection", "connection in"=w453) -> ()  [unwired: 3 in, 6 out]
            }
            frame True {
            }
          }
        }
        n330 = TCP Close Connection(connection ID=w324, error in (no error)=w326) -> (error out=w325:errorcluster)  [unwired: 1 in, 1 out]
        n331 = call <vilib>:"Clear Errors.vi"("error in (no error)"=w325) -> ()  [unwired: 5 in, 2 out]
      }
    }
    n332 = Wait (ms)(milliseconds to wait=u32 500) -> ()  [unwired: 1 out]
    n333 = local read "Saiu?"() -> (w320:bool)
  }
  n334 = Obtain Notifier(name (unnamed)="BlocoSinais", notification data type=T3 {"SinaisAlta"=[], "SinaisBaixa"=[], "NumBloco"=0} ("output cluster")) -> (notifier out=w8:refnum<notifier>)  [unwired: 2 in, 2 out]
  n335 = while {
    shift-right: [w461] -> _
    shift-left: variant[] [] -> [w463]
    tunnel: w10 -> [_]
    tunnel: [w458] -> w13
    tunnel: w8 -> [w457]
    i -> [w460]
    stop <- w458 stop-if-true
    # "Loop de geração de sinais\n1. Para cada canal, gera o sinal de acordo com o tipo e os parâmetros configurados\n2. Obtém o estado final da última iteração\n3. Gera o waveform e o estado final da geração de acordo com o tipo de sinal\n4. Se sinalizado pelo ResetCanais, reinicia o estado de todos os sinais gerados\n5. Mostra o sinal do canal selecionado nos gráficos"
    # "LOOP DE GERAÇÃO DE SINAIS DINÂMICOS"
    n336 = local read "Habilitar"() -> (w459:bool)
    n337 = case shown="True" w459 {
      tunnel: w463 -> [w464 w477]
      tunnel: [w464 w475] -> w461
      tunnel: w460 -> [_ w472]
      tunnel: w457 -> [_ w465]
      frame False {
      }
      frame True {
        # "4."
        n338 = local read "TxAmostragem"() -> (w470:dbl)
        n339 = local read "DadosCanais"() -> (w478:T2[])
        n340 = for {
          tunnel: w478 -> [w499] mode=indexing
          tunnel: w477 -> [w498]
          tunnel: [w493] -> w476 mode=indexing
          tunnel: w470 -> [w492]
          tunnel: [w491] -> w473 mode=indexing
          i -> [w497]
          # "3."
          # "2."
          # "1."
          n341 = Unbundle By Name(w499) -> ("Tipo"=w496:T1, "params"=w495:variant)
          n342 = Index Array(array=w498, index=w497) -> (element=w494:variant)
          n343 = case shown="\"AM\"" w496 {
            tunnel: w495 -> [w504 w509 w514 w519 w522 w529 w534 _]
            tunnel: w494 -> [w503 w507 w512 w517 w520 w527 w532 _]
            tunnel: [w502 w505 w510 w515 w524 w525 w530 _] -> w493
            tunnel: w492 -> [w501 w508 w513 w518 w521 w528 w533 _]
            tunnel: [w500 w506 w511 w516 w523 w526 w531 _] -> w491
            frame "Ruído" {
              n344 = call "GeraSinalRuido.vi"("params"=w504, "Tx Aquisicao"=w501, "estadoIn"=w503) -> ("sinal"=w502:waveform(dbl), "estadoOut"=w500:variant)  [unwired: 15 in]
            }
            frame "Fasor" {
              n345 = call "GeraSinalFasor.vi"("params"=w509, "Tx Aquisicao"=w508, "estadoIn"=w507) -> ("sinal"=w505:waveform(dbl), "estadoOut"=w506:variant)  [unwired: 15 in]
            }
            frame "Senóide" {
              n346 = call "GeraSinalSenoide.vi"("params"=w514, "Tx Aquisicao"=w513, "estadoIn"=w512) -> ("sinal"=w510:waveform(dbl), "estadoOut"=w511:variant)  [unwired: 15 in]
            }
            frame "Composto" {
              n347 = call "GeraSinalComposto.vi"("params"=w519, "Tx Aquisicao"=w518, "estadoIn"=w517) -> ("sinal"=w515:waveform(dbl), "estadoOut"=w516:variant)  [unwired: 15 in]
            }
            frame "AM" {
              n348 = call "GeraSinalAM.vi"("params"=w522, "Tx Aquisicao"=w521, "estadoIn"=w520) -> ("sinal"=w524:waveform(dbl), "estadoOut"=w523:variant)  [unwired: 15 in]
            }
            frame "Proximidade" {
              n349 = call "GeraSinalProximeter.vi"("params"=w529, "Tx Aquisicao"=w528, "estadoIn"=w527) -> ("sinal"=w525:waveform(dbl), "estadoOut"=w526:variant)  [unwired: 15 in]
            }
            frame "Entreferro" {
              n350 = call "GeraSinalEntreferro.vi"("params"=w534, "Tx Aquisicao"=w533, "estadoIn"=w532) -> ("sinal"=w530:waveform(dbl), "estadoOut"=w531:variant)  [unwired: 15 in]
            }
            frame Default {
            }
          }
        }
        n351 = local read "TxAmostragemBaixa"() -> (w469:dbl)
        n352 = local read "ResetCanais"() -> (w468:bool)
        n353 = flat-sequence {
          tunnel: w476 -> [w480]
          tunnel: w472 -> [w484]
          tunnel: [w484] -> w471
          tunnel: w470 -> [w483]
          tunnel: w469 -> [w482]
          tunnel: w468 -> [w481]
          tunnel: [w480] -> w467
          tunnel: [w479] -> w466
          tunnel: w471 -> [w487]
          tunnel: w467 -> [w489]
          tunnel: w466 -> [w488]
          tunnel: w465 -> [w486]
          frame #0 {
            n354 = call "ProcessaSinalBaixa.vi"("Sinais"=w480, "TxAmostragem"=w483, "TxAmostragemBaixa"=w482, "Reset"=w481) -> ("SinaisBaixa"=w479:waveform(dbl)[])  [unwired: 15 in]
            "SinaisBaixa" <- w479
            "Sinais" <- w480
          }
          frame #1 {
            n355 = Bundle(w489, "SinaisBaixa"=w488, w487) -> (w485:T17)  [unwired: 1 in]
            n356 = Send Notification(notification=w485, notifier=w486) -> ()  [unwired: 1 in, 2 out]
            "NumBloco" <- w487
          }
        }
        n357 = Select(t=variant[] [] ("f"), s=w468, f=w473) -> (s? t:f=w475:variant[])
        n358 = case shown="True" w468 {
          frame False {
          }
          frame True {
            n359 = local write "ResetCanais"(FALSE ("ResetCanais")) -> ()
          }
        }
      }
    }
    n360 = Wait (ms)(milliseconds to wait=u32 1000) -> ()  [unwired: 1 out]
    n361 = local read "Saiu?"() -> (w458:bool)
  }
  n362 = local read "BlocoBaixaEnviado"() -> (w1:i32)
  n363 = Increment(x=w1) -> (x+1=→"BlocoBaixaEnviado":i32)
  n364 = while {
    stop <- w540 stop-if-true
    n365 = local read "SinaisBaixa"() -> (w538:waveform(dbl)[])
    n366 = local read "Sinais"() -> (w537:waveform(dbl)[])
    n367 = local read "Canais"() -> (w544:i32[])
    n368 = Select(t=w538, s="Vizualizar Baixa", f=w537) -> (s? t:f=w542:waveform(dbl)[])
    n369 = for {
      tunnel: w542 -> [w549]
      tunnel: [w546] -> w539 mode=indexing
      tunnel: [w547] -> w535 mode=indexing
      tunnel: w544 -> [w548] mode=indexing
      tunnel: "Ver Fase" -> [w545]
      # "5."
      n370 = Index Array(array=w549, index=w548) -> (element=w547:waveform(dbl))
      n371 = call "FFTSemDC.vi"("wfm"=w547, "Fase"=w545) -> ("FFT"=w546:cluster{"f0":dbl, "df":dbl, "magnitude":dbl[]})  [unwired: 17 in]
    }
    "Tempo" <- w535
    "Frequência" <- w539
    n372 = Wait (ms)(milliseconds to wait=u32 1000) -> ()  [unwired: 1 out]
    n373 = local read "Saiu?"() -> (w540:bool)
  }
  n374 = flat-sequence {
    tunnel: w14 -> [_]
    tunnel: w13 -> [_]
    tunnel: w12 -> [_]
    tunnel: w11 -> [_]
    frame #0 {
      # "FINALIZA敲O"
      n375 = property class="App"() -> ("App.Kind"=w550:T18)  [unwired: 2 in, 2 out]
      n376 = case shown="\"Run Time System\"" w550 {
        frame Default {
        }
        frame "Run Time System" {
          n377 = Quit LabVIEW() -> ()  [unwired: 1 in]
        }
      }
    }
  }
